vi "Rotation_Equals.vi"(9 "other ROTATION":T1={"VALUE"=0.0, "COS"=1.0, "SIN"=0.0} {"SIN" format="%13.4f"; "COS" format="%13.4f"; "VALUE" format="%13.4f"}, 11 "in ROTATION":T1={"VALUE"=0.0, "COS"=1.0, "SIN"=0.0} {"SIN" format="%13.4f"; "COS" format="%13.4f"; "VALUE" format="%13.4f"}) -> (3 "Equals":bool)   [LabVIEW 2019, in "Trajectory_Library.lvlib"]
doc: "Checks equality between this Rotation2d and another object.\n\nParameters:\n - in ROTATION - This Rotation data structure\n - other ROTATION - The other Rotation to compare\n\nReturns:\n - equals - Whether the two objects are equal or not."
uses:
  Trajectory_Library.lvlib
  ROTATION2D.ctl
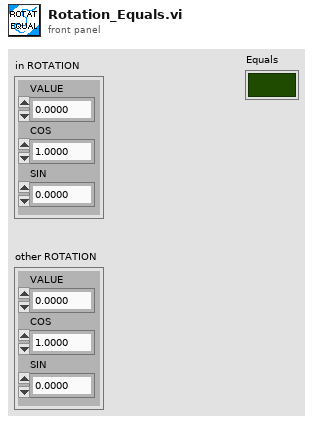
[diagram p1: front panel]
types:
  T1 = typedef "Trajectory_Library.lvlib/ROTATION2D.ctl" = cluster{"VALUE":dbl, "COS":dbl, "SIN":dbl}
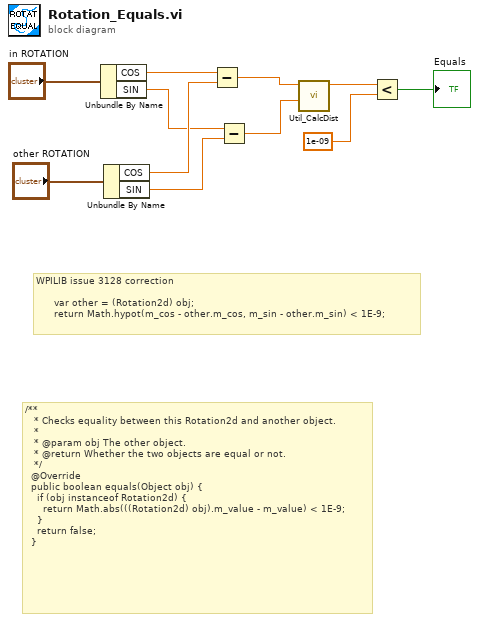
[diagram p0: block diagram]
diagram:
  # "WPILIB issue 3128 correction \n\n      var other = (Rotation2d) obj;\n      return Math.hypot(m_cos - other.m_cos, m_sin - other.m_sin) < 1E-9;"
  # "/**\n   * Checks equality between this Rotation2d and another object.\n   *\n   * @param obj The other object.\n   * @return Whether the two objects are equal or not.\n   */\n  @Override\n  public boolean equals(Object obj) {\n    if (obj instanceof Rotation2d) {\n      return Math.abs(((Rotation2d) obj).m_value - m_value) < 1E-9;\n    }\n    return false;\n  }"
  n1 = Unbundle By Name("in ROTATION") -> ("COS"=w7:dbl, "SIN"=w5:dbl)
  n2 = Unbundle By Name("other ROTATION") -> ("COS"=w6:dbl, "SIN"=w4:dbl)
  n3 = Subtract(x=w7, y=w6) -> (x-y=w3:dbl)
  n4 = Subtract(x=w5, y=w4) -> (x-y=w2:dbl)
  n5 = call "Util_CalcDist.vi"("Y"=w2, "X"=w3) -> ("DIST"=w1:dbl)  [unwired: 9 in]
  n6 = Less?(x=w1, y=1e-09) -> (x < y?=→"Equals":bool)
